vi "CreateIntegerMatrix.vi"(1 "colunas":i32, 2 "linhas":i32) -> (0 "2D matrix":T1)   [LabVIEW 2019]
uses:
  <vilib>/Analysis/Matrix/Datatypes/RealMatrix.ctl
  <vilib>/Analysis/Matrix/NI_Matrix.lvlib
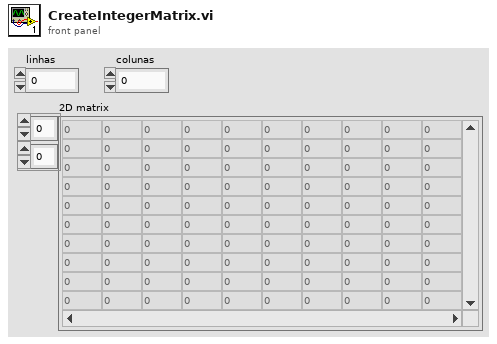
[diagram p1: front panel]
types:
  T1 = typedef "NI_Matrix.lvlib/RealMatrix.ctl" = dbl[][]
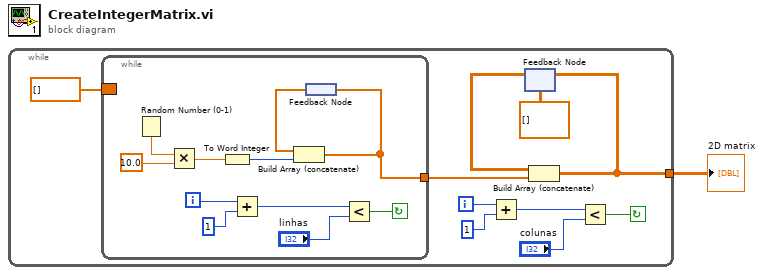
[diagram p0: block diagram]
diagram:
  n1 = while {
    tunnel: [w6] -> w1
    i -> [w5]
    stop <- w11 continue-if-true
    n2 = while {
      tunnel: [w18] -> w9
      border: dbl[] [] -> [_]
      i -> [w14]
      stop <- w19 continue-if-true
      n3 = Random Number (0-1)() -> (number: 0 to 1=w22:dbl)
      n4 = Multiply(x=w22, y=10.0) -> (x*y=w17:dbl)
      n5 = To Word Integer(number=w17) -> (16bit integer=w16:i16)
      n6 = Add(x=w14, y=1) -> (x+y=w12:i32)
      n7 = feedback #1() -> (w20:dbl[])
      n8 = Build Array (concatenate)(w20, w16) -> (w18:dbl[])
      n9 = feedback-in #1(w18) -> ()
      n10 = Less?(x=w12, y="linhas") -> (x < y?=w19:bool)
    }
    n11 = Add(x=w5, y=1) -> (x+y=w3:i32)
    n12 = feedback #2(T1 [] ("Real Matrix")) -> (w10:T1)
    n13 = Build Array (concatenate)(w10, w9) -> (w6:T1)
    n14 = feedback-in #2(w6) -> ()
    n15 = Less?(x=w3, y="colunas") -> (x < y?=w11:bool)
  }
  "2D matrix" <- w1
